vi "BMark_MainWindow.vi"() -> ()   [LabVIEW 2018]
uses:
  controls/BMark_UI Data.ctl
  <vilib>/addons/analyzer/_analyzerctrls.llb/VIAnCtl Analysis App Info.ctl
  controls/BMark_Bookmark Data.ctl
  controls/BMark_VI_Identifier.ctl
  <vilib>/event_ctls.llb/eventvkey.ctl
  <vilib>/Utility/miscctls.llb/LVNodeAndColumnTypeDef.ctl
  <vilib>/Utility/miscctls.llb/LVRectTypeDef.ctl
  globals/BMark_User Visible Strings.vi
  support/Message Queue/BMark_Message Queue.lvlib
  support/User Event - Stop/BMark_User Event - Stop.lvlib
panel:
  in  "Scope":u16(ring)
  in  "More information link":bool
  out "Warning glyph":bool
  in  "Group":enum32{"Group by Tag", "Group by VI"}(radio)
  in  "Tree":string(tree)
  in  "Help":bool
  in  "Close":bool
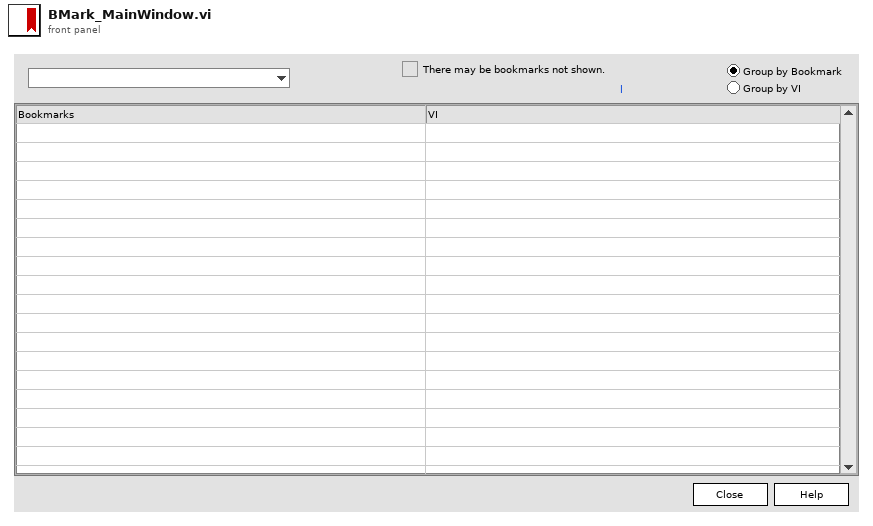
[diagram p1: front panel]
types:
  T1 = typedef "BMark_UI Data.ctl" = cluster{"Projects":refnum<vi>, "Tree":refnum<vi>, "GroupBy":refnum<vi>, "Warning glyph":refnum<vi>, "More information":refnum<vi>, "Front Panel":refnum<vi>, "GroupByVI":bool, "all projects":T2[], "bookmarks":T3[], "App Info":T2, "TopLeft Tag":string, "Collapsed Tags":string[], "Reset BM Cache?":bool}
  T2 = typedef "VIAnCtl Analysis App Info.ctl" = cluster{"Project Name":string, "Target Name":string}
  T3 = typedef "BMark_Bookmark Data.ctl" = cluster{"bookmark tag":string, "full text":string, "bookmark ref":i32, "VI display name":string, "VI identifier":T4}
  T4 = typedef "BMark_VI_Identifier.ctl" = cluster{"Name":string, "Path":path, "App Info":T2}
  T5 = typedef "BMark_Message Queue.lvlib/All Message Queues.ctl" = cluster{"UI":refnum<queue>}
  T6 = typedef "eventvkey.ctl" = enum16{"ASCII", "Enter", "Return", "Shift", "Ctrl", "Alt", "Cmd", "Opt", "Caps", "NumLock", "Clear", "Break", "Up", "Down", "Left", "Right", "Insert", "Delete", "Home", "End", "PageUp", "PageDown", "Escape", "Help", "Pause", "ScrollLock", "F1", "F2", "F3", "F4", "F5", "F6", "F7", "F8", "F9", "F10", "F11", "F12", "F13", "F14", "F15", "F16", "F17", "F18", "F19", "F20", "F21", "F22", "F23", "F24", "Play", "VolumeUp", "VolumeDown", "Mute", "Two Byte Char"}
  T7 = typedef "LVRectTypeDef.ctl" = cluster{"Left":i16, "Top":i16, "Right":i16, "Bottom":i16}
  T8 = enum8{"Enabled", "Disabled", "Disabled and Grayed Out"}
  T9 = typedef "LVNodeAndColumnTypeDef.ctl" = cluster{"Node":string, "Column":i32}
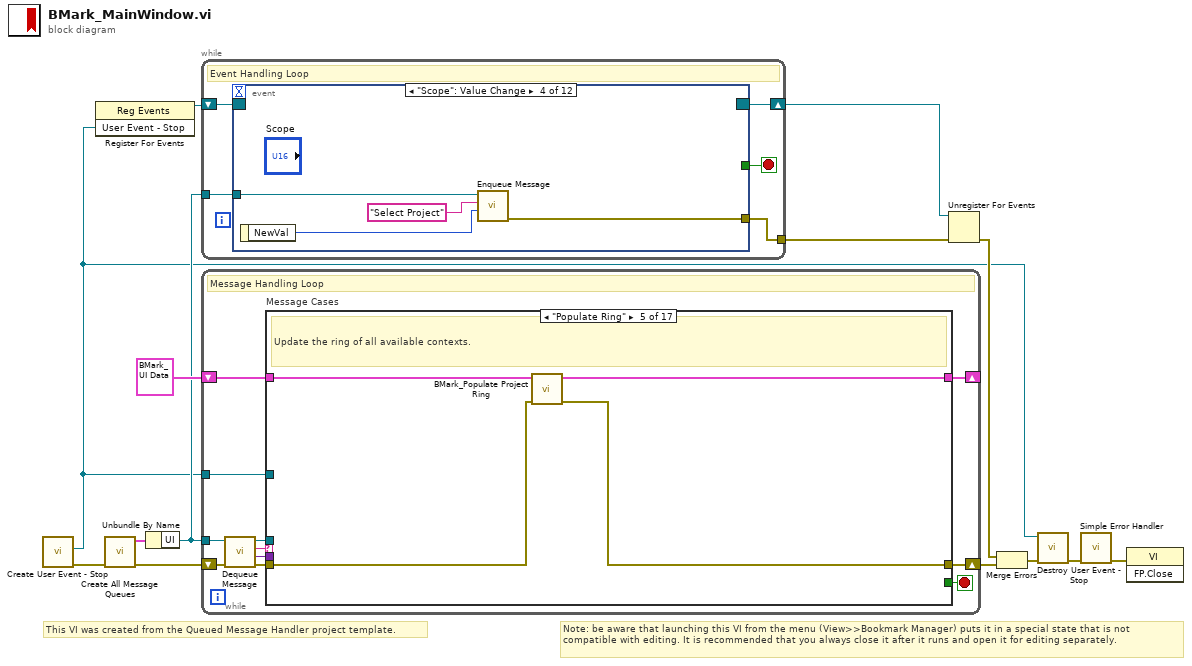
[diagram p0: block diagram]
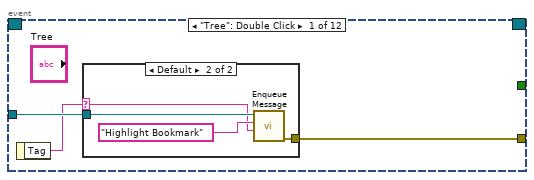
[diagram p2: hidden frame]
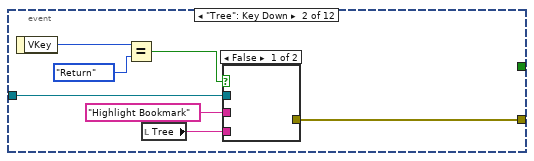
[diagram p4: hidden frame]
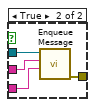
[diagram p5: hidden frame]
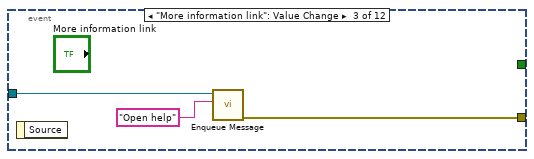
[diagram p6: hidden frame]
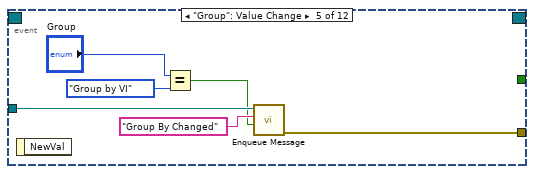
[diagram p7: hidden frame]
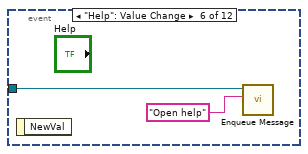
[diagram p8: hidden frame]
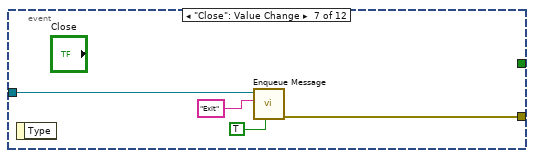
[diagram p9: hidden frame]
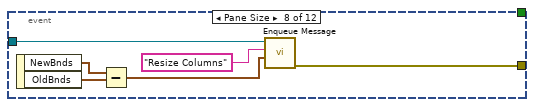
[diagram p10: hidden frame]
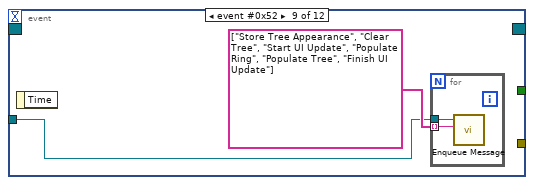
[diagram p11: hidden frame]
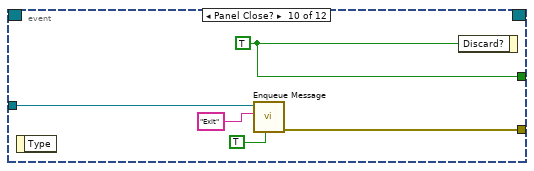
[diagram p12: hidden frame]
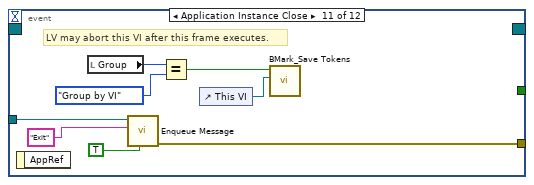
[diagram p13: hidden frame]
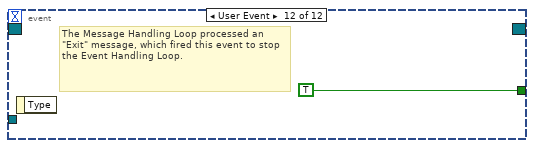
[diagram p14: hidden frame]
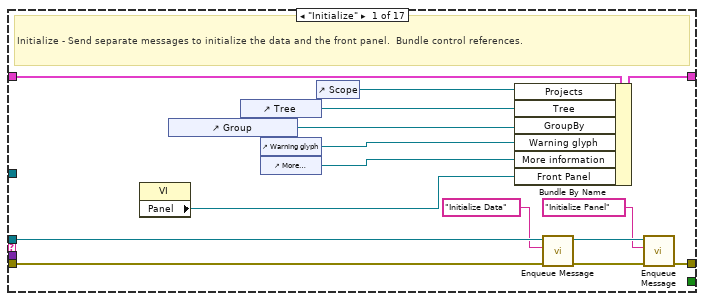
[diagram p15: hidden frame]
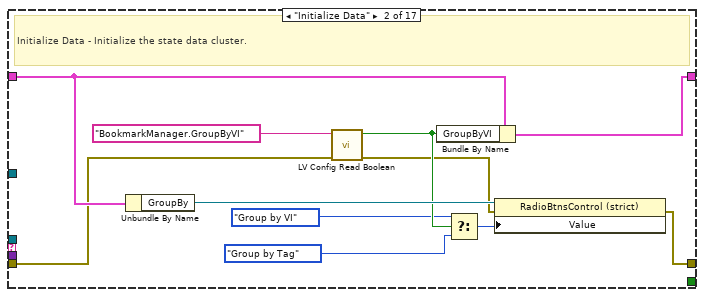
[diagram p16: hidden frame]
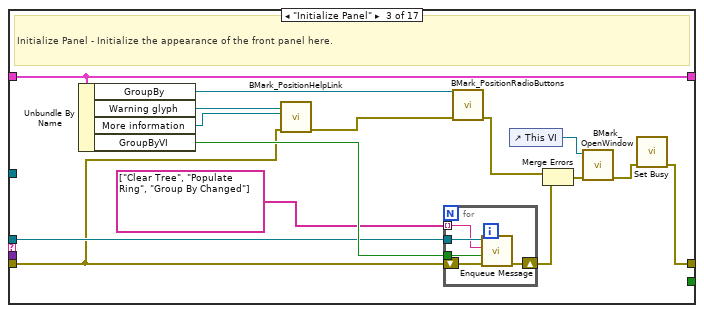
[diagram p17: hidden frame]
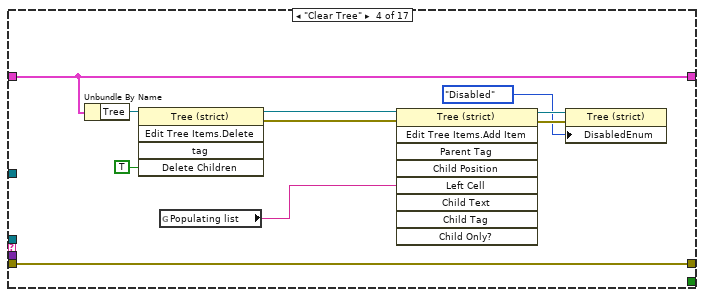
[diagram p18: hidden frame]
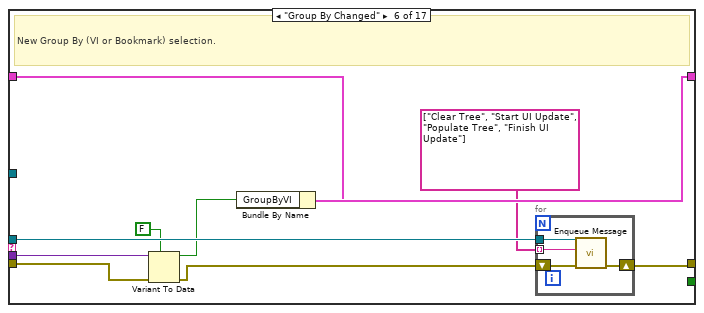
[diagram p19: hidden frame]
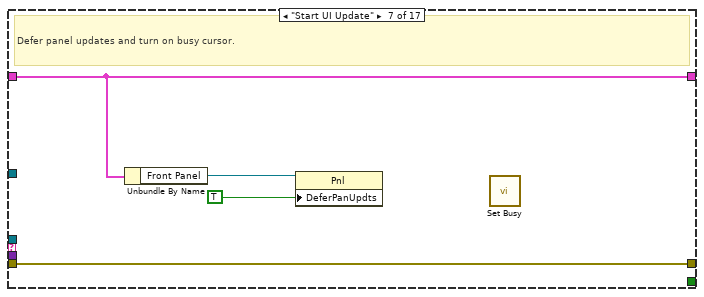
[diagram p20: hidden frame]
diagram:
  # "Note: be aware that launching this VI from the menu (View>>Bookmark Manager) puts it in a special state that is not compatible with editing. It is recommended that you always close it after it runs and open it for editing separately."
  # "This VI was created from the Queued Message Handler project template."
  n1 = call <resource>:"Create User Event - Stop.vi"() -> ("error out"=w9:errorcluster, "User Event - Stop"=w1:refnum<user-event>)  [unwired: 10 in]
  n2 = register-events(w1) -> (reference out=w2:refnum<event-registration>)  [unwired: 2 in, 1 out]
  n3 = call <resource>:"Create All Message Queues.vi"("error in (no error)"=w9) -> ("error out"=w5:errorcluster, "Message Queues out"=w6:T5)  [unwired: 9 in]
  n4 = Unbundle By Name(w6) -> ("UI"=w8:refnum<queue>)
  n5 = while {
    tunnel: w8 -> [w19]
    tunnel: [w18] -> w12
    shift-right: [w16] -> w13
    shift-left: w2 -> [w17]
    stop <- w15 stop-if-true
    # "Event Handling Loop"
    n6 = event shown="[3] \"Scope\": Value Change" {
      selector: w17 -> [_ _ _ _ _ _ _ _ _ _ _ _]
      dyn-events: [_ _ _ _ _ _ _ _ _ _ _ _] -> w16
      timeout: _ -> [_ _ _ _ _ _ _ _ _ _ _ _]
      tunnel: [_ _ _ _ _ _ _ _ _ w71 _ TRUE ("Discard?")] -> w15
      tunnel: w19 -> [w22 w33 w40 w44 w50 w51 w56 w61 w63 w70 w79 _]
      tunnel: [w21 w32 w38 w43 w49 _ w55 w60 _ w69 w78 _] -> w18
      event "Tree": Double Click {
        n7 = event-data() -> ("Tag"=w20:string)  [unwired: 1 in]
        n8 = case shown="Default" w20 {
          selector: w20 -> [_ w23]
          tunnel: w22 -> [_ w26]
          tunnel: [_ w25] -> w21
          frame "" {
          }
          frame Default {
            n9 = call <resource>:"Enqueue Message.vi"("Message Data"=w23, "Message"="Highlight Bookmark", "Message Queue"=w26) -> ("error out"=w25:errorcluster)  [unwired: 7 in, 1 out]
          }
        }
      }
      event "Tree": Key Down {
        n10 = event-data() -> ("VKey"=w29:T6)  [unwired: 1 in]
        n11 = Equal?(x=w29, y=eventvkey."Return") -> (x = y?=w30:bool)
        n12 = local read "Tree"() -> (w27:string)
        n13 = case shown="False" w30 {
          tunnel: w33 -> [_ w37]
          tunnel: [_ w36] -> w32
          tunnel: "Highlight Bookmark" ("Message") -> [_ w35]
          tunnel: w27 -> [_ w34]
          frame False {
          }
          frame True {
            n14 = call <resource>:"Enqueue Message.vi"("Message Data"=w34, "Message"=w35, "Message Queue"=w37) -> ("error out"=w36:errorcluster)  [unwired: 7 in, 1 out]
          }
        }
      }
      event "More information link": Value Change {
        n15 = event-data() -> ()  [unwired: 1 in, 1 out]
        n16 = call <resource>:"Enqueue Message.vi"("Message"="Open help", "Message Queue"=w40) -> ("error out"=w38:errorcluster)  [unwired: 8 in, 1 out]
      }
      event "Scope": Value Change {
        n17 = event-data() -> ("NewVal"=w41:u16)  [unwired: 1 in]
        n18 = call <resource>:"Enqueue Message.vi"("Message Data"=w41, "Message"="Select Project", "Message Queue"=w44) -> ("error out"=w43:errorcluster)  [unwired: 7 in, 1 out]
      }
      event "Group": Value Change {
        n19 = event-data() -> ()  [unwired: 1 in, 1 out]
        n20 = Equal?(x="Group", y=enum32{"Group by Tag", "Group by VI"}."Group by VI" ("GroupBy")) -> (x = y?=w45:bool)
        n21 = call <resource>:"Enqueue Message.vi"("Message Data"=w45, "Message"="Group By Changed", "Message Queue"=w50) -> ("error out"=w49:errorcluster)  [unwired: 7 in, 1 out]
      }
      event "Help": Value Change {
        n22 = event-data() -> ()  [unwired: 1 in, 1 out]
        n23 = call <resource>:"Enqueue Message.vi"("Message"="Open help", "Message Queue"=w51) -> ()  [unwired: 8 in, 2 out]
      }
      event "Close": Value Change {
        n24 = event-data() -> ()  [unwired: 1 in, 1 out]
        n25 = call <resource>:"Enqueue Message.vi"("Priority Message? (F)"=TRUE, "Message"="Exit", "Message Queue"=w56) -> ("error out"=w55:errorcluster)  [unwired: 7 in, 1 out]
      }
      event Pane Size {
        n26 = event-data() -> ("NewBnds"=w59:T7, "OldBnds"=w58:T7)  [unwired: 1 in]
        n27 = Subtract(x=w59, y=w58) -> (x-y=w57:T7)
        n28 = call <resource>:"Enqueue Message.vi"("Message Data"=w57, "Message"="Resize Columns", "Message Queue"=w61) -> ("error out"=w60:errorcluster)  [unwired: 7 in, 1 out]
      }
      event event #0x52 {
        n29 = event-data() -> ()  [unwired: 1 in, 1 out]
        n30 = for {
          tunnel: w63 -> [w66]
          tunnel: string[] ["Store Tree Appearance", "Clear Tree", "Start UI Update", "Populate Ring", "Populate Tree", "Finish UI Update"] -> [w65] mode=indexing
          n31 = call <resource>:"Enqueue Message.vi"("Message"=w65, "Message Queue"=w66) -> ()  [unwired: 8 in, 2 out]
        }
      }
      event Panel Close? {
        w71 = TRUE ("Discard?")
        n32 = event-data() -> ()  [unwired: 1 in, 1 out]
        n33 = call <resource>:"Enqueue Message.vi"("Priority Message? (F)"=TRUE, "Message"="Exit", "Message Queue"=w70) -> ("error out"=w69:errorcluster)  [unwired: 7 in, 1 out]
        n34 = event-data("Discard?"=w71) -> ()  [unwired: 1 in, 1 out]
      }
      event Application Instance Close {
        # "LV may abort this VI after this frame executes."
        n35 = event-data() -> ()  [unwired: 1 in, 1 out]
        n36 = local read "Group"() -> (w74:enum32{"Group by Tag", "Group by VI"})
        n37 = call <resource>:"Enqueue Message.vi"("Priority Message? (F)"=TRUE, "Message"="Exit", "Message Queue"=w79) -> ("error out"=w78:errorcluster)  [unwired: 7 in, 1 out]
        n38 = Equal?(x=w74, y=enum32{"Group by Tag", "Group by VI"}."Group by VI" ("GroupBy")) -> (x = y?=w72:bool)
        n39 = control-ref of="This VI"() -> (w75:refnum<vi>)
        n40 = call "BMark_Save Tokens.vi"("reference"=w75, "GroupByVI"=w72) -> ()  [unwired: 10 in]
      }
      event User Event {
        # "The Message Handling Loop processed an \"Exit\" message, which fired this event to stop the Event Handling Loop."
        n41 = event-data() -> ()  [unwired: 1 in, 1 out]
      }
    }
  }
  n42 = while {
    tunnel: w8 -> [w81]
    shift-right: [w90] -> _
    shift-left: T1 {"Projects"=refnum, "Tree"=refnum, "GroupBy"=refnum, "Warning glyph"=refnum, "More information"=refnum, "Front Panel"=refnum, "GroupByVI"=FALSE, "all projects"=[], "bookmarks"=[], "App Info"={"Project Name"="", "Target Name"=""}, "TopLeft Tag"="", "Collapsed Tags"=[], "Reset BM Cache?"=FALSE} ("Data Cluster") -> [w91]
    tunnel: w1 -> [w87]
    shift-right: [w88] -> w7
    shift-left: w5 -> [w86]
    stop <- w89 stop-if-true
    # "Message Handling Loop"
    n43 = call <resource>:"Dequeue Message.vi"("error in (no error)"=w86, "Message Queue"=w81) -> ("error out"=w85:errorcluster, "Message Data"=w83:variant, "Message"=w84:string, "dup Message Queue"=w82:refnum<queue>)  [unwired: 6 in]
    n44 = case "Message Cases" shown="\"Populate Ring\"" w84 {
      selector: w84 -> [_ _ _ _ _ _ _ _ _ _ _ _ _ _ _ _ w305]
      tunnel: w82 -> [w102 _ w121 _ _ w158 _ _ w192 _ _ w253 _ _ _ w300 _]
      tunnel: w85 -> [w105 w109 w120 w147 w151 w161 w169 w178 w199 w200 w234 w259 w268 w276 w290 w296 _]
      tunnel: [w106 w107 w122 w147 w150 w154 w169 w178 w189 w200 w228 w252 w264 w276 w289 w297 w303] -> w88
      tunnel: w91 -> [w99 w114 w132 w146 w149 w155 w166 w177 w195 w214 w238 w256 w273 w275 w286 w293 w306]
      tunnel: [w98 w116 w132 w146 w148 w159 w166 w176 w193 w203 w238 w255 w273 w275 w286 w293 w306] -> w90
      tunnel: [_ _ _ _ _ _ _ _ _ _ _ _ _ _ _ TRUE _] -> w89
      tunnel: w83 -> [_ _ _ _ _ w160 _ _ _ _ w236 w258 w269 _ w288 _ _]
      tunnel: w87 -> [_ _ _ _ _ _ _ _ _ _ _ _ _ _ _ w295 _]
      frame "Initialize" {
        # "Initialize - Send separate messages to initialize the data and the front panel.  Bundle control references."
        n45 = property class="VI"() -> ("Panel"=w92:refnum<vi>)  [unwired: 2 in, 2 out]
        n46 = control-ref of="Group"() -> (w95:refnum<vi>)
        n47 = control-ref of="Tree"() -> (w96:refnum<vi>)
        n48 = control-ref of="Warning glyph"() -> (w94:refnum<vi>)
        n49 = control-ref of="More information link"() -> (w93:refnum<vi>)
        n50 = control-ref of="Scope"() -> (w97:refnum<vi>)
        n51 = Bundle By Name(cluster=w99, "Projects"=w97, "Tree"=w96, "GroupBy"=w95, "Warning glyph"=w94, "More information"=w93, "Front Panel"=w92) -> (w98:T1)
        n52 = call <resource>:"Enqueue Message.vi"("error in (no error)"=w105, "Message"="Initialize Data", "Message Queue"=w102) -> ("error out"=w104:errorcluster, "dup Message Queue"=w103:refnum<queue>)  [unwired: 7 in]
        n53 = call <resource>:"Enqueue Message.vi"("error in (no error)"=w104, "Message"="Initialize Panel", "Message Queue"=w103) -> ("error out"=w106:errorcluster)  [unwired: 7 in, 1 out]
      }
      frame "Initialize Data" {
        # "Initialize Data - Initialize the state data cluster."
        n54 = Unbundle By Name(w114) -> ("GroupBy"=w115:refnum<vi>)
        n55 = call <resource>:"LV Config Read Boolean.vi"("error in"=w109, "key"="BookmarkManager.GroupByVI") -> ("error out"=w108:errorcluster, "value"=w113:bool)  [unwired: 3 in, 1 out]
        n56 = Bundle By Name(cluster=w114, "GroupByVI"=w113) -> (w116:T1)
        n57 = Select(t=enum32{"Group by Tag", "Group by VI"}."Group by VI" ("GroupBy"), s=w113, f=enum32{"Group by Tag", "Group by VI"}."Group by Tag" ("GroupBy")) -> (s? t:f=w110:enum32{"Group by Tag", "Group by VI"})
        n58 = property class="RadioBtnsControl (strict)"(reference=w115, error in=w108, "Value"=w110) -> (error out=w107:errorcluster)  [unwired: 1 out]
      }
      frame "Initialize Panel" {
        # "Initialize Panel - Initialize the appearance of the front panel here."
        n59 = Unbundle By Name(w132) -> ("GroupBy"=w131:refnum<vi>, "Warning glyph"=w129:refnum<vi>, "More information"=w128:refnum<vi>, "GroupByVI"=w130:bool)
        n60 = call "BMark_PositionHelpLink.vi"("error in (no error)"=w120, "More information"=w128, "Warning glyph"=w129) -> ("error out"=w127:errorcluster)  [unwired: 8 in]
        n61 = for {
          tunnel: w130 -> [w137]
          tunnel: w121 -> [w135]
          tunnel: string[] ["Clear Tree", "Populate Ring", "Group By Changed"] -> [w133] mode=indexing
          shift-right: [w136] -> w125
          shift-left: w120 -> [w134]
          n62 = call <resource>:"Enqueue Message.vi"("error in (no error)"=w134, "Message Data"=w137, "Message"=w133, "Message Queue"=w135) -> ("error out"=w136:errorcluster)  [unwired: 6 in, 1 out]
        }
        n63 = call "BMark_PositionRadioButtons.vi"("error in (no error)"=w127, "RadioButtonsControl in"=w131) -> ("error out"=w126:errorcluster)  [unwired: 9 in]
        n64 = control-ref of="This VI"() -> (w118:refnum<vi>)
        n65 = Merge Errors(w126, w125) -> (w124:errorcluster)
        n66 = call "BMark_OpenWindow.vi"("error in (no error)"=w124, "Bookmark manager window reference"=w118) -> ("error out"=w123:errorcluster)  [unwired: 7 in, 2 out]
        n67 = call <vilib>:"Set Busy.vi"("error in (no error)"=w123) -> ("error out"=w122:errorcluster)  [unwired: 9 in, 1 out]
      }
      frame "Clear Tree" {
        n68 = Unbundle By Name(w146) -> ("Tree"=w145:refnum<vi>)
        n69 = invoke class="Tree (strict)" method="Edit Tree Items.Delete"(reference=w145, "Delete Children"=TRUE ("Delete Children?")) -> (reference out=w143:refnum<vi>, error out=w142:errorcluster)  [unwired: 3 in, 3 out]
        n70 = global read "BMark_User Visible Strings.vi" "Populating list"() -> (w141:string)
        n71 = invoke class="Tree (strict)" method="Edit Tree Items.Add Item"(reference=w143, error in=w142, "Left Cell"=w141) -> (reference out=w140:refnum<vi>, error out=w139:errorcluster)  [unwired: 6 in, 7 out]
        n72 = property class="Tree (strict)"(reference=w140, error in=w139, "DisabledEnum"=T8."Disabled" ("Disabled")) -> ()  [unwired: 2 out]
      }
      frame "Populate Ring" {
        # "Update the ring of all available contexts."
        n73 = call "BMark_Populate Project Ring.vi"("error in (no error)"=w151, "Data Cluster in"=w149) -> ("error out"=w150:errorcluster, "Data Cluster out"=w148:T1)  [unwired: 8 in]
      }
      frame "Group By Changed" {
        # "New Group By (VI or Bookmark) selection."
        n74 = Variant To Data(error in=w161, type=FALSE, Variant=w160) -> (data=w156:bool, error out=w152:errorcluster)
        n75 = Bundle By Name(cluster=w155, "GroupByVI"=w156) -> (w159:T1)
        n76 = for {
          tunnel: w158 -> [w165]
          tunnel: string[] ["Clear Tree", "Start UI Update", "Populate Tree", "Finish UI Update"] -> [w164] mode=indexing
          shift-right: [w163] -> w154
          shift-left: w152 -> [w162]
          n77 = call <resource>:"Enqueue Message.vi"("error in (no error)"=w162, "Message"=w164, "Message Queue"=w165) -> ("error out"=w163:errorcluster)  [unwired: 7 in, 1 out]
        }
      }
      frame "Start UI Update" {
        # "Defer panel updates and turn on busy cursor."
        n78 = Unbundle By Name(w166) -> ("Front Panel"=w167:refnum<vi>)
        n79 = property class="Pnl"(reference=w167, "DeferPanUpdts"=TRUE ("Defer Panel Updates")) -> ()  [unwired: 1 in, 2 out]
        n80 = call <vilib>:"Set Busy.vi"() -> ()  [unwired: 10 in, 2 out]
      }
      frame "Store Tree Appearance" {
        # "Ignore any errors that may occur here. Being unable to store the tree appearance is not critical to the operation of the Bookmark Manager, and as such, should not generate an error that would shut down the entire UI."
        # "Store the scroll position and expanded items of the tree to restore later."
        n81 = Unbundle By Name(w177) -> ("Tree"=w173:refnum<vi>)
        n82 = property class="Tree (strict)"(reference=w173) -> (reference out=w171:refnum<vi>, "TopLeft"=w175:T9, "All Tags"=w172:string[])  [unwired: 1 in, 1 out]
        n83 = for {
          tunnel: w172 -> [w183] mode=indexing
          tunnel: w171 -> [w184]
          tunnel: [w183] -> w170 mode=indexing if=w179
          # "Item is collapsed if indent = 0 and not open"
          n84 = property class="Tree (strict)"(reference=w184, "Active Item Tag"=w183) -> ("Indent Level"=w181:i32, "Open?"=w180:bool)  [unwired: 1 in, 2 out]
          n85 = Equal To 0?(x=w181) -> (x = 0?=w182:bool)
          n86 = Compound Arithmetic op=AND(w182, invert w180) -> (w179:bool)
        }
        n87 = Unbundle By Name(w175) -> ("Node"=w174:string)
        n88 = Bundle By Name(cluster=w177, "TopLeft Tag"=w174, "Collapsed Tags"=w170) -> (w176:T1)
      }
      frame "Populate Tree" {
        # "Update the tree of bookmarks. Turn off the Reset BM Cache? flag so the cache for the current project can be used until the user changes the project ring."
        n89 = Unbundle By Name(w195) -> ("App Info"=w186:T2, "Reset BM Cache?"=w185:bool, "Tree"=w197:refnum<vi>, "GroupByVI"=w196:bool)
        n90 = call "BMark_Get Bookmarks.vi"("error in (no error)"=w199, "Reset BM Cache?"=w185, "App Info"=w186) -> ("error out"=w198:errorcluster, "possible undisplayed bookmarks"=w190:bool, "bookmarks"=w194:T3[])  [unwired: 5 in, 1 out]
        n91 = call "BMark_Create Tree.vi"("error in (no error)"=w198, "GroupByVI"=w196, "TreeRef"=w197, "Bookmark info"=w194) -> ("error out"=w188:errorcluster)  [unwired: 7 in]
        n92 = Bundle By Name(cluster=w195, "Reset BM Cache?"=FALSE, "bookmarks"=w194) -> (w193:T1)
        n93 = call <resource>:"Enqueue Message.vi"("error in (no error)"=w188, "Message Data"=w190, "Message"="Show/Hide Help Link", "Message Queue"=w192) -> ("error out"=w189:errorcluster)  [unwired: 6 in, 1 out]
      }
      frame "Finish UI Update" {
        # "Ignore any errors that may occur here. Being unable to restore the tree appearance is not critical to the operation of the Bookmark Manager, and as such, should not generate an error that would shut down the entire UI."
        # "Restore collapsed items (if any), restore the previous scroll position (if there is one), then undefer panel updates."
        n94 = Unbundle By Name(w214) -> ("Tree"=w205:refnum<vi>, "Collapsed Tags"=w204:string[], "TopLeft Tag"=w212:string, "Front Panel"=w213:refnum<vi>)
        n95 = case shown="Default" w212 {
          selector: w212 -> [_ w223]
          tunnel: w205 -> [w219 w222]
          tunnel: [w218 w221] -> w209
          tunnel: [w216 w223] -> w207
          tunnel: w204 -> [_ w220]
          frame "" {
            n96 = property class="Tree (strict)"(reference=w219) -> (reference out=w218:refnum<vi>, "All Tags"=w217:string[])  [unwired: 1 in, 1 out]
            n97 = Index Array(array=w217) -> (element=w216:string)  [unwired: 1 in]
          }
          frame Default {
            n98 = for {
              shift-right: [w226] -> w221
              shift-left: w222 -> [w227]
              tunnel: w220 -> [w225] mode=indexing
              n99 = property class="Tree (strict)"(reference=w227, "Active Item Tag"=w225, "Open?"=FALSE) -> (reference out=w226:refnum<vi>)  [unwired: 1 in, 1 out]
            }
          }
        }
        n100 = Bundle By Name(cluster=T9 {"Node"="", "Column"=0} ("Top Left Visible Cell"), "Node"=w207) -> (w206:T9)
        n101 = property class="Tree (strict)"(reference=w209, "TopLeft"=w206) -> (error out=w211:errorcluster)  [unwired: 1 in, 1 out]
        n102 = call <vilib>:"Clear Errors.vi"("error in (no error)"=w211) -> ("error out"=w210:errorcluster)  [unwired: 5 in, 1 out]
        n103 = Bundle By Name(cluster=w214, "TopLeft Tag"="", "Collapsed Tags"=string[] []) -> (w203:T1)
        n104 = property class="Pnl"(reference=w213, error in=w210, "DeferPanUpdts"=FALSE ("Defer Panel Updates")) -> ()  [unwired: 2 out]
        n105 = call <vilib>:"Unset Busy.vi"() -> ()  [unwired: 11 in, 1 out]
      }
      frame "Highlight Bookmark" {
        # "Highlight the bookmark."
        n106 = Unbundle By Name(w238) -> ("bookmarks"=w229:T3[], "Tree"=w237:refnum<vi>)
        n107 = Variant To Data(error in=w234, type="", Variant=w236) -> (data=w230:string, error out=w233:errorcluster)
        n108 = property class="Tree (strict)"(reference=w237, error in=w233, "Active Item Tag"=w230) -> (error out=w232:errorcluster, "Indent Level"=w239:i32)  [unwired: 1 out]
        n109 = Greater Than 0?(x=w239) -> (x > 0?=w231:bool)
        n110 = case shown="True" w231 {
          tunnel: w232 -> [w240 w246]
          tunnel: [w240 w243] -> w228
          tunnel: w230 -> [_ w245]
          tunnel: w229 -> [_ w244]
          frame False {
          }
          frame True {
            n111 = call "BMark_Highlight Bookmark.vi"("error in (no error)"=w246, "bookmarks"=w244, "tag"=w245) -> ("error out"=w242:errorcluster)  [unwired: 8 in]
            n112 = call <vilib>:"Simple Error Handler.vi"("error in (no error)"=w242) -> ("error out"=w241:errorcluster)  [unwired: 4 in, 4 out]
            n113 = call <vilib>:"Clear Errors.vi"("error in (no error)"=w241) -> ("error out"=w243:errorcluster)  [unwired: 5 in, 1 out]
          }
        }
      }
      frame "Select Project" {
        # "New project (or Main Application Instance) selected. Set the Reset BM Cache? flag so the Get Bookmarks VI can retrieve a fresh list of bookmarks for the newly-selected project."
        n114 = Unbundle By Name(w256) -> ("all projects"=w250:T2[])
        n115 = Variant To Data(error in=w259, type=u16 0 ("Projects"), Variant=w258) -> (data=w249:u16, error out=w254:errorcluster)
        n116 = call "BMark_Get App From Ring Selection.vi"("all projects"=w250, "Projects"=w249) -> ("App Info"=w248:T2)  [unwired: 9 in]
        n117 = Bundle By Name(cluster=w256, "Reset BM Cache?"=TRUE, "App Info"=w248) -> (w255:T1)
        n118 = for {
          tunnel: w253 -> [w262]
          shift-right: [w261] -> w252
          shift-left: w254 -> [w263]
          tunnel: string[] ["Clear Tree", "Start UI Update", "Populate Tree", "Finish UI Update"] -> [w260] mode=indexing
          n119 = call <resource>:"Enqueue Message.vi"("error in (no error)"=w263, "Message"=w260, "Message Queue"=w262) -> ("error out"=w261:errorcluster)  [unwired: 7 in, 1 out]
        }
      }
      frame "Show/Hide Help Link" {
        n120 = Unbundle By Name(w273) -> ("Warning glyph"=w272:refnum<vi>, "More information"=w271:refnum<vi>)
        n121 = Variant To Data(error in=w268, type=FALSE ("Visible"), Variant=w269) -> (data=w266:bool, error out=w267:errorcluster)
        n122 = property class="Bool (strict)"(reference=w271, error in=w267, "Visible"=w266) -> (error out=w265:errorcluster)  [unwired: 1 out]
        n123 = property class="Bool (strict)"(reference=w272, error in=w265, "Visible"=w266) -> (error out=w264:errorcluster)  [unwired: 1 out]
      }
      frame "Open help" {
        n124 = call <helpdir>:"_LaunchHelp.vi"("HTML filename"="bkmk_manager_moreinfo.html") -> ()  [unwired: 6 in, 1 out]
      }
      frame "Resize Columns" {
        # "This code makes the second column of the tree \"fill\" the available space so that additional columns are never visible. Note: this doesn't work correctly if the user resizes the columns."
        n125 = Unbundle By Name(w286) -> ("Tree"=w285:refnum<vi>)
        n126 = Variant To Data(error in=w290, type=T7 {"Left"=0, "Top"=0, "Right"=0, "Bottom"=0} ("NewBnds"), Variant=w288) -> (data=w282:T7, error out=w289:errorcluster)
        n127 = Unbundle By Name(w282) -> ("Right"=w281:i16, "Left"=w280:i16)
        n128 = property class="Tree (strict)"(reference=w285, "ActiveColNum"=1 ("Active Cell:Active Column Number")) -> (reference out=w278:refnum<vi>, "Width"=w283:i32)  [unwired: 1 in, 1 out]
        n129 = Subtract(x=w281, y=w280) -> (x-y=w279:i16)
        n130 = Add(x=w283, y=w279) -> (x+y=w277:i32)
        n131 = property class="Tree (strict)"(reference=w278, "Width"=w277) -> ()  [unwired: 1 in, 2 out]
      }
      frame "Exit" {
        # "Stop the VI"
        # "Release the message queue reference"
        # "Close the Bookmark Manager window. Note that this case may not execute when quitting LabVIEW. Refer to the Application Instance Close frame in the Event Handling Loop."
        n132 = Unbundle By Name(w293) -> ("GroupByVI"=w292:bool)
        n133 = control-ref of="This VI"() -> (w291:refnum<vi>)
        n134 = call <resource>:"Fire User Event - Stop.vi"("User Event - Stop"=w295) -> ("error out"=w294:errorcluster)  [unwired: 10 in]
        n135 = call "BMark_Save Tokens.vi"("reference"=w291, "GroupByVI"=w292) -> ()  [unwired: 10 in]
        n136 = Release Queue(queue=w300, error in (no error)=w296) -> (error out=w298:errorcluster)  [unwired: 1 in, 2 out]
        n137 = Merge Errors(w294, w298) -> (w297:errorcluster)
      }
      frame Default {
        # "'Default' case only runs if there is a message that isn't defined in any of the other cases.  Output a programming error."
        n138 = global read "BMark_User Visible Strings.vi" "unknown message error"() -> (w301:string)
        n139 = Format Into String(format string=w301, w305) -> (resulting string=w302:string)  [unwired: 2 in, 1 out]
        n140 = call <vilib>:"Error Cluster From Error Code.vi"("error message (\"\")"=w302, "error code (0)"=1) -> ("error out"=w303:errorcluster)  [unwired: 7 in]
      }
    }
  }
  n141 = Unregister For Events(event registration refnum=w13, error in=w12) -> (error out=w11:errorcluster)
  n142 = Merge Errors(w11, w7) -> (w10:errorcluster)
  n143 = call <resource>:"Destroy User Event - Stop.vi"("error in (no error)"=w10, "User Event - Stop"=w1) -> ("error out"=w4:errorcluster)  [unwired: 9 in]
  n144 = call <vilib>:"Simple Error Handler.vi"("error in (no error)"=w4) -> ("error out"=w3:errorcluster)  [unwired: 4 in, 4 out]
  n145 = invoke class="VI" method="FP.Close"(error in=w3) -> ()  [unwired: 2 in, 3 out]
